vi "getAllStateNames.vi"(8 "error in (no error)":errorcluster, 11 "Channel in":refnum<class "Channel.lvclass">) -> (0 "error out":errorcluster, 2 "state_names":string[](array[string]), 3 "Channel out":refnum<class "Channel.lvclass">)   [LabVIEW 2009, in "Tools.lvlib" / "DatabaseHelpers.lvlib" / "Channel.lvclass"]
uses:
  Channel.lvclass
  Channel.lvclass/Channel.ctl
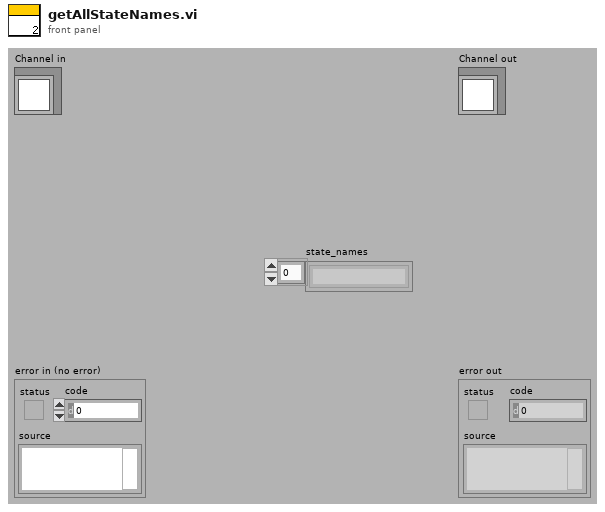
[diagram p1: front panel]
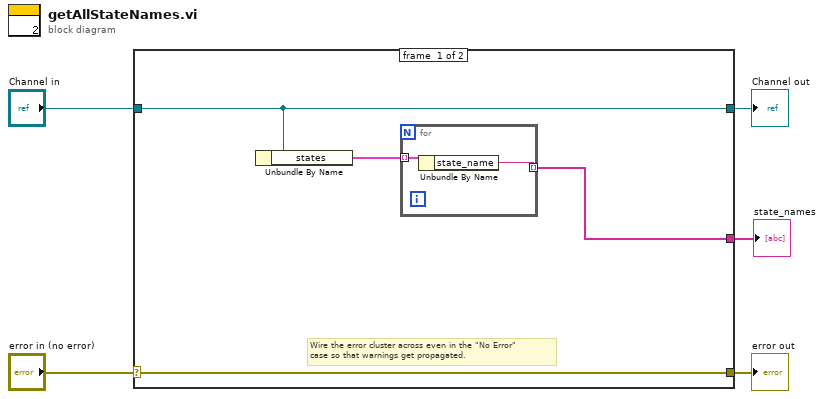
[diagram p0: block diagram]
diagram:
  n1 = case shown="No Error" "error in (no error)" {
    selector: "error in (no error)" -> [w9 w13]
    tunnel: [w9 w13] -> w4
    tunnel: [w8 w12] -> w2
    tunnel: "Channel in" -> [w8 w12]
    tunnel: [w6 _] -> w1
    frame #0 {
      # "Wire the error cluster across even in the \"No Error\"\ncase so that warnings get propagated."
      n2 = Unbundle By Name(w8) -> ("states"=w7:cluster{"state_name":string, "value":string}[])
      n3 = for {
        tunnel: w7 -> [w11] mode=indexing
        tunnel: [w10] -> w6 mode=indexing
        n4 = Unbundle By Name(w11) -> ("state_name"=w10:string)
      }
    }
    frame #1 {
    }
  }
  "error out" <- w4
  "Channel out" <- w2
  "state_names" <- w1
